vi "initHandler.vi"(8 "error in (no error)":errorcluster, 9 "Name":string, 10 "Level":T1(ring), 11 "Handler.UserEvent.Console in":refnum<class "Handler.UserEvent.Console.lvclass">) -> (0 "error out":errorcluster, 3 "Handler.UserEvent.Console out":refnum<class "Handler.UserEvent.Console.lvclass">)   [LabVIEW 2017, in "Error Log.lvlib" / "Handler.UserEvent.Console.lvclass"]
uses:
  Handler.UserEvent.Console.lvclass
  Handler.UserEvent.Console.lvclass/Handler.UserEvent.Console.ctl
  Handler.UserEvent/Handler.UserEvent.lvclass
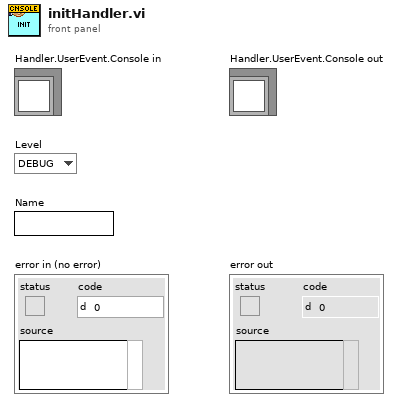
[diagram p1: front panel]
types:
  T1 = enum16{"DEBUG", "INFO", "WARNING", "ERROR", "CRITICAL"}
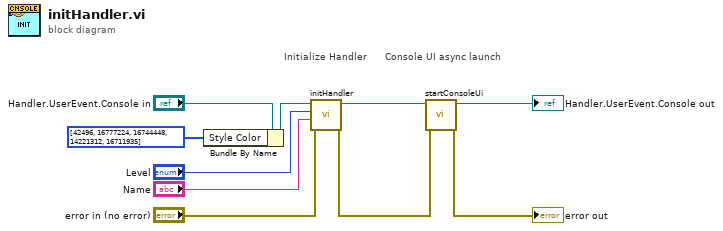
[diagram p0: block diagram]
diagram:
  # "Console UI async launch"
  # "Initialize Handler"
  n1 = Bundle By Name(cluster="Handler.UserEvent.Console in", "Style Color"=u32[] [42496, 16777224, 16744448, 14221312, 16711935]) -> (w2:refnum<class "Handler.UserEvent.Console.lvclass">)
  n2 = call-parent "initHandler.vi"("error in (no error)"="error in (no error)", "Name"="Name", "Level"="Level", "Handler.UserEvent in"=w2) -> ("error out"=w6:errorcluster, "Handler.UserEvent out"=w5:refnum<class "Handler.UserEvent.Console.lvclass">)  [unwired: 6 in]
  n3 = call-dynamic "startConsoleUi.vi"("error in (no error)"=w6, "Handler.UserEvent.Console in"=w5) -> ("error out"=→"error out":errorcluster, "Handler.UserEvent.Console out"=→"Handler.UserEvent.Console out":refnum<class "Handler.UserEvent.Console.lvclass">)  [unwired: 8 in]
